vi "仪器电源管理.vi"() -> ()   [LabVIEW 2016, in "环境动力监测库.lvlib" / "G电源管理库.lvlib"]
uses:
  <vilib>/Utility/miscctls.llb/LVPointTypeDef.ctl
panel:
  in  "电源控制":T1
  in  "副屏看门狗启用":u16(ring) caption="副屏看门狗启用：" items=["关闭", "打开"]
  in  "副屏看门狗设置":u16 caption="副屏看门狗设置："
  out "副屏看门狗计时":u16 caption="副屏看门狗计时："
  in  "主屏看门狗启用":u16(ring) caption="主屏看门狗启用：" items=["关闭", "打开"]
  in  "主屏看门狗设置":u16 caption="主屏看门狗设置："
  out "主屏看门狗计时":u16 caption="主屏看门狗计时："
  # "仪器电源管理"
  # "s"
  # "s"
  # "s"
  # "s"
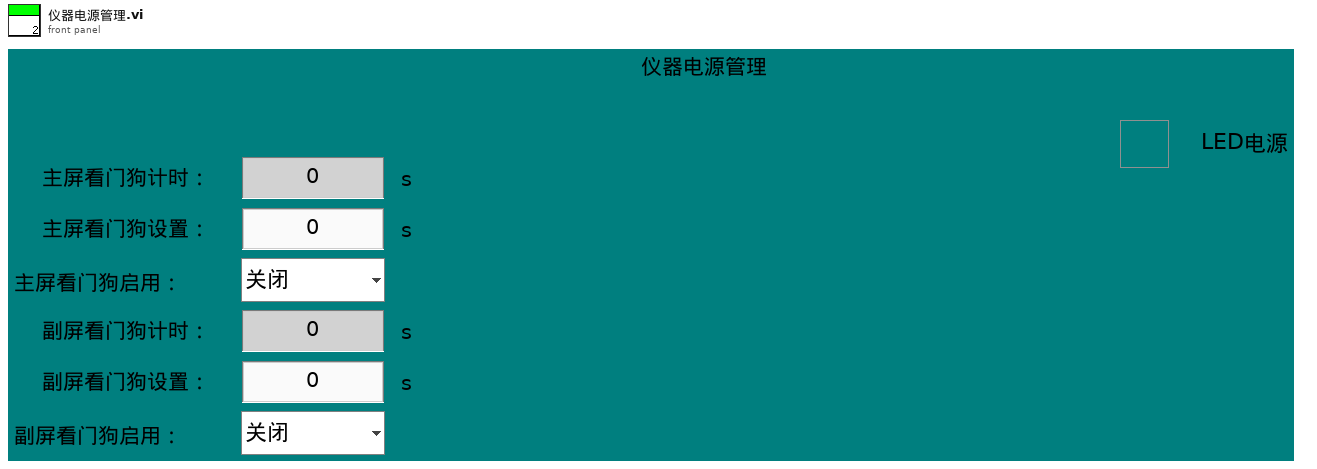
[diagram p1: front panel]
types:
  T1 = cluster{"氨氮电源":bool, "总磷电源":bool, "总氮电源":bool, "多参数电源":bool, "CODMn电源":bool, "CODCr电源":bool, "LED电源":bool}
  T2 = typedef "LVPointTypeDef.ctl" = cluster{"Horizontal":i16, "Vertical":i16}
  T3 = cluster{"采配水启用":bool, "CODMn启用":bool, "CODcr启用":bool, "氨氮启用":bool, "总磷启用":bool, "质控单元启用":bool, "流量计启用":bool, "电源管理启用":bool, "其他启用":bool, "多参数启用":bool, "超标留样启用":bool, "总氮启用":bool, "运行模式":enum16{"维护模式", "常规模式", "应急模式", "质控模式"}}
  T4 = cluster{"状态":cluster{"R0":i16, "R1":i16, "R2":i16, "R3":i16, "R4":i16, "R5":i16, "R6":i16, "R7":i16, "R8":i16, "R9":i16, "R10":i16, "R11":i16, "R12":i16, "R13":i16, "R14":i16, "R15":i16, "R16":i16, "R17":i16, "R18":i16, "R19":i16, "R20":i16, "R21":i16, "R22":i16, "R23":i16, "R24":i16, "R25":i16, "R26":i16, "R27":i16, "R28":i16, "R29":i16, "R30":i16, "R31":i16, "R32":i16, "R33":i16, "R34":i16, "R35":i16, "R36":i16, "R37":i16, "R38":i16, "R39":i16}, "输入状态":bool[], "输出状态":bool[], "参数设置":cluster{"R100":i16, "R101":i16, "R102":i16, "R103":i16, "R104":i16, "R105":i16, "R106":i16, "R107":i16, "R108":i16, "R109":i16, "R110":i16, "R111":i16, "R112":i16, "R113":i16, "R114":i16, "R115":i16, "R116":i16, "R117":i16, "R118":i16, "R119":i16, "R120":i16, "R121":i16, "R122":i16, "R123":i16}, "转换值":cluster{"AD0":sgl, "AD1":sgl, "AD2":sgl, "AD3":sgl, "AD4":sgl, "AD5":sgl}}
  T5 = cluster{"R100":i16, "R101":i16, "R102":i16, "R103":i16, "R104":i16, "R105":i16, "R106":i16, "R107":i16, "R108":i16, "R109":i16, "R110":i16, "R111":i16, "R112":i16, "R113":i16, "R114":i16, "R115":i16, "R116":i16, "R117":i16, "R118":i16, "R119":i16, "R120":i16, "R121":i16, "R122":i16, "R123":i16}
  T6 = cluster{"R0":i16, "R1":i16, "R2":i16, "R3":i16, "R4":i16, "R5":i16, "R6":i16, "R7":i16, "R8":i16, "R9":i16, "R10":i16, "R11":i16, "R12":i16, "R13":i16, "R14":i16, "R15":i16, "R16":i16, "R17":i16, "R18":i16, "R19":i16, "R20":i16, "R21":i16, "R22":i16, "R23":i16, "R24":i16, "R25":i16, "R26":i16, "R27":i16, "R28":i16, "R29":i16, "R30":i16, "R31":i16, "R32":i16, "R33":i16, "R34":i16, "R35":i16, "R36":i16, "R37":i16, "R38":i16, "R39":i16}
  T7 = cluster{"命令":string, "数据":cluster{"starting address":u16, "holding register values":u16[]}}
  T8 = cluster{"命令":string, "数据":cluster{"starting address":u16, "holding register value":u16}}
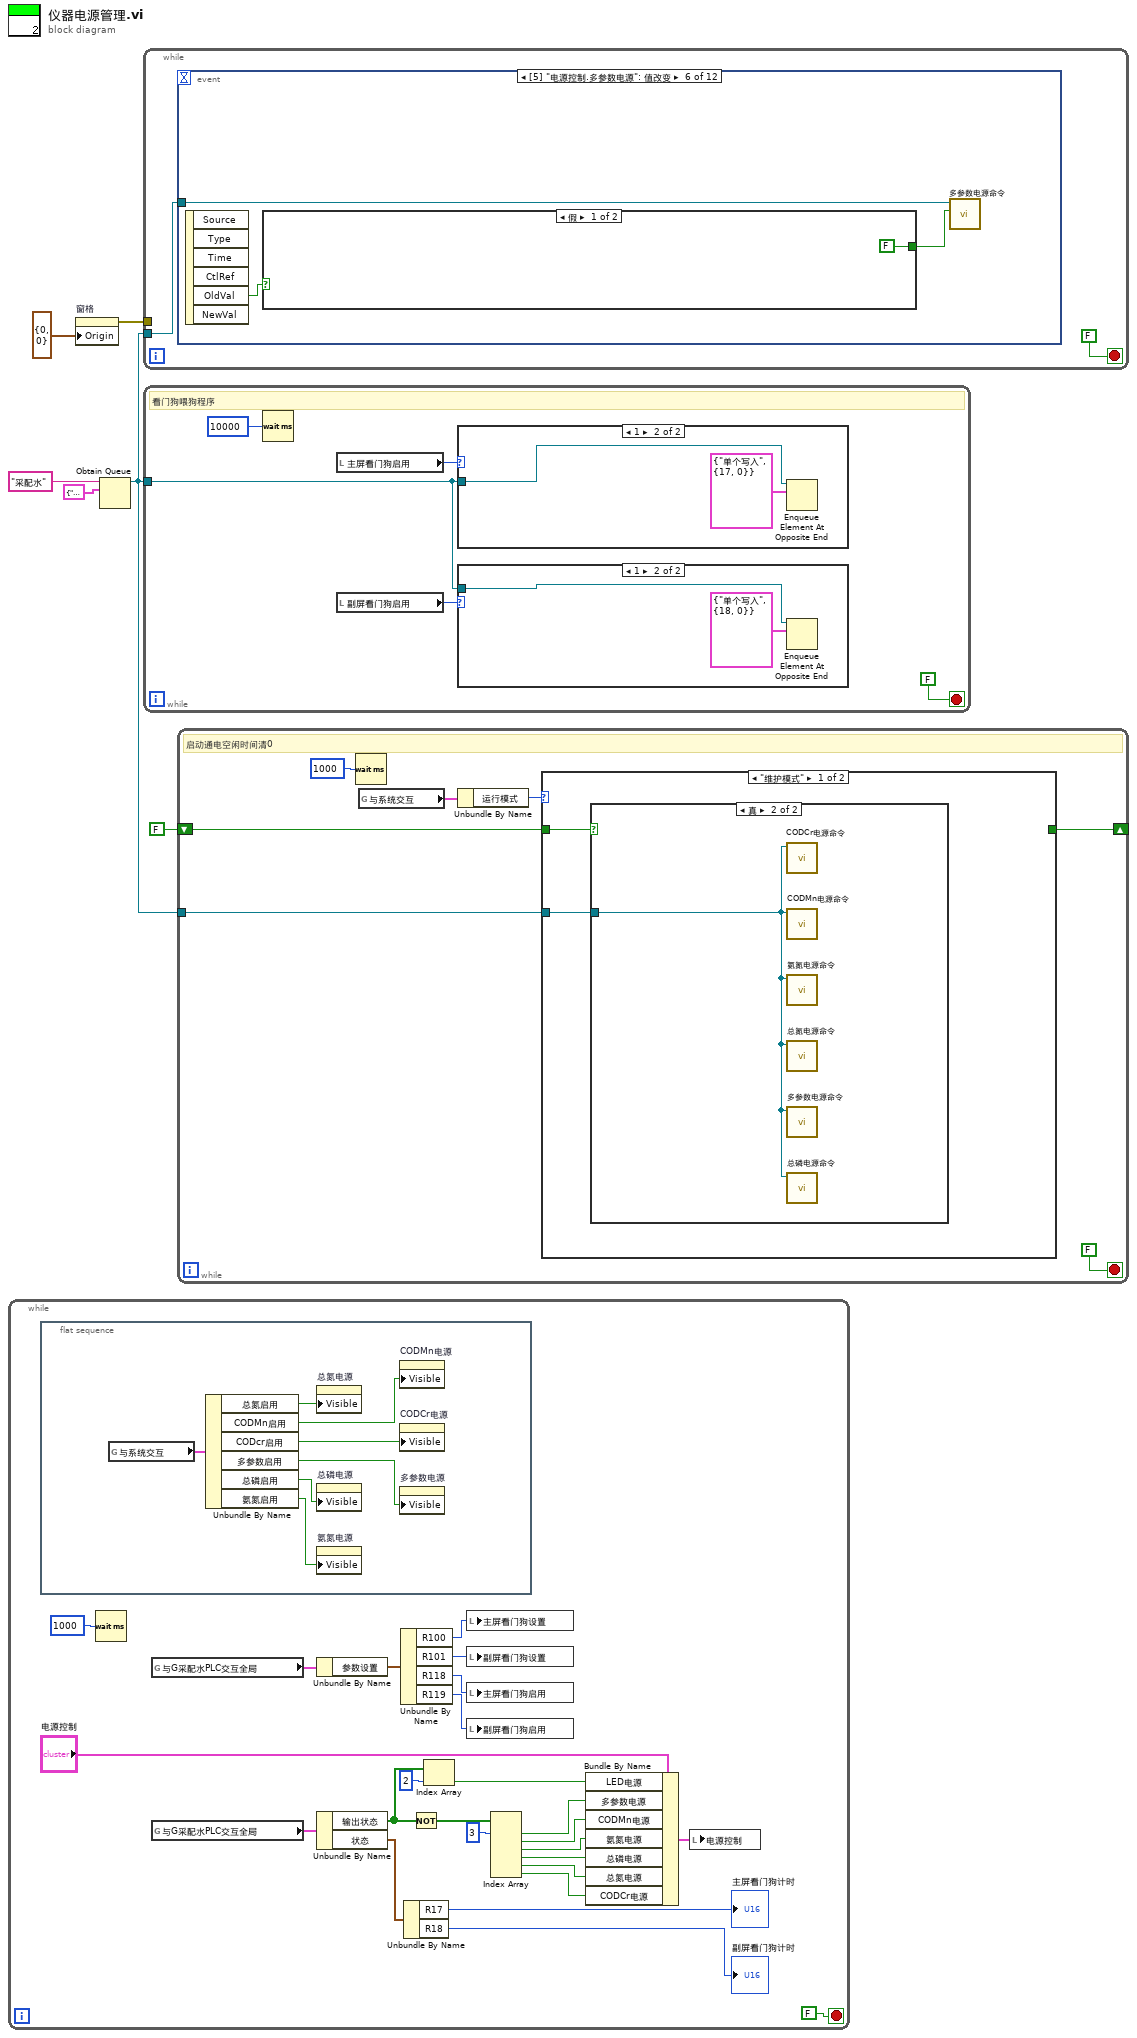
[diagram p0: block diagram]
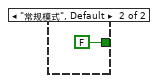
[diagram p5: hidden frame]
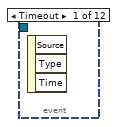
[diagram p6: hidden frame]
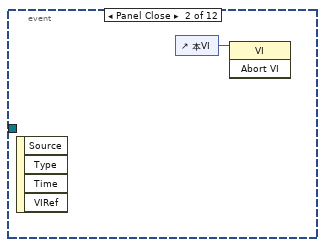
[diagram p7: hidden frame]
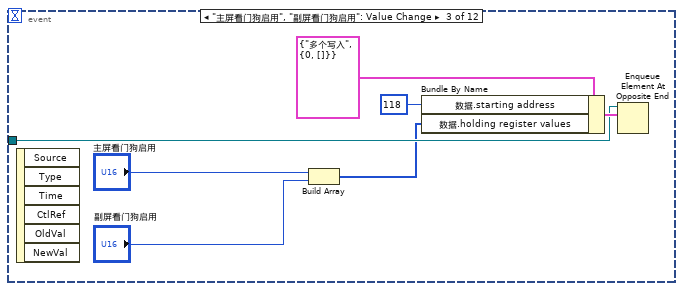
[diagram p8: hidden frame]
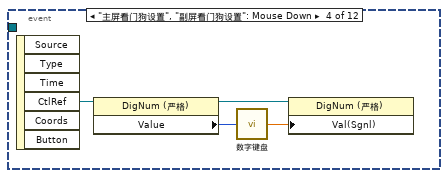
[diagram p9: hidden frame]
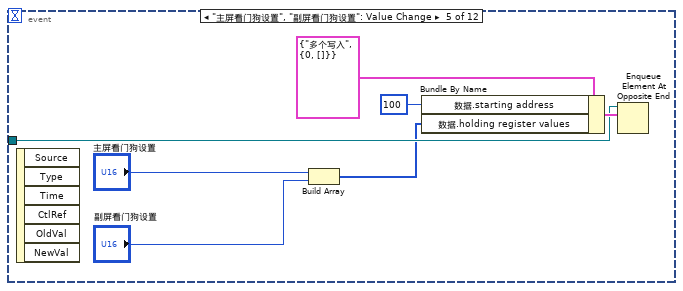
[diagram p10: hidden frame]
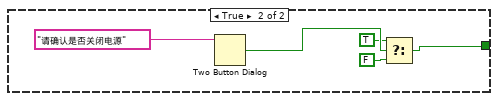
[diagram p11: hidden frame]
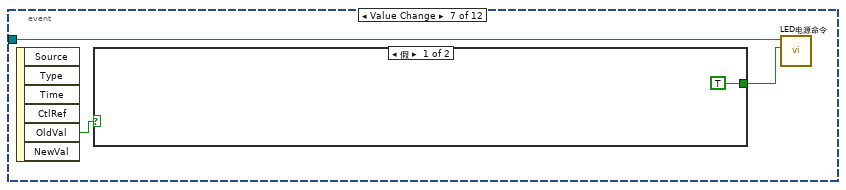
[diagram p12: hidden frame]
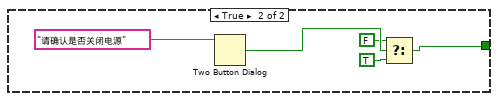
[diagram p13: hidden frame]
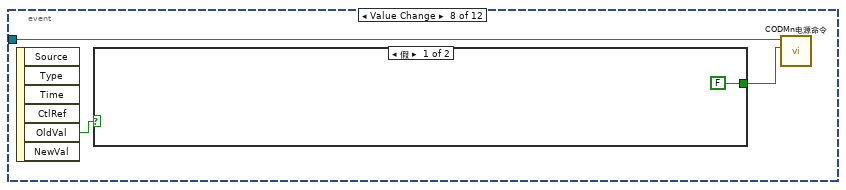
[diagram p14: hidden frame]
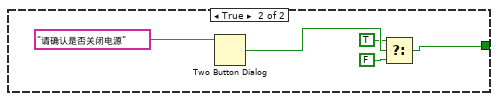
[diagram p15: hidden frame]
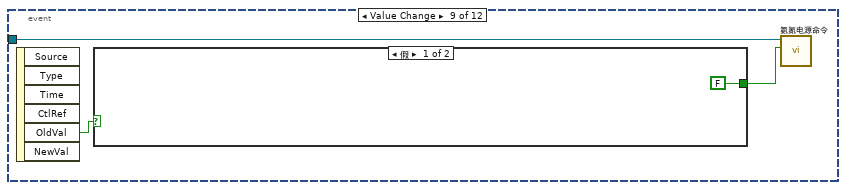
[diagram p16: hidden frame]
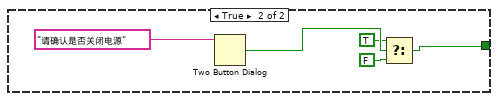
[diagram p17: hidden frame]
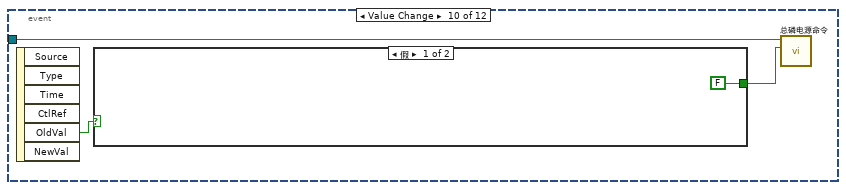
[diagram p18: hidden frame]
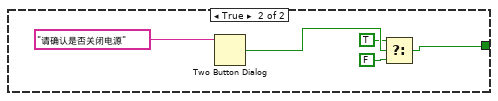
[diagram p19: hidden frame]
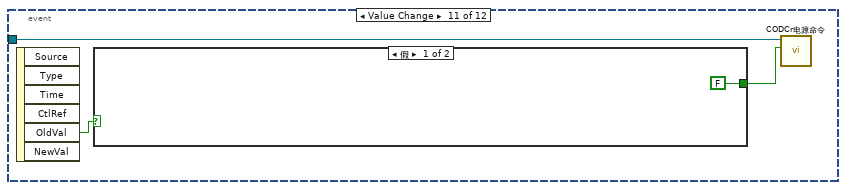
[diagram p20: hidden frame]
diagram:
  n1 = while {
    stop <- FALSE stop-if-true
    n2 = flat-sequence {
      frame #0 {
        n3 = global read "外部交互全局变量.vi" "与系统交互"() -> (w38:T3)
        n4 = Unbundle By Name(w38) -> ("总氮启用"=w37:bool, "CODMn启用"=w36:bool, "CODcr启用"=w32:bool, "多参数启用"=w33:bool, "总磷启用"=w34:bool, "氨氮启用"=w35:bool)
        n5 = property on="总氮电源" class="Bool (严格)"("Visible"=w37) -> ()  [unwired: 2 in, 2 out]
        n6 = property on="总磷电源" class="Bool (严格)"("Visible"=w34) -> ()  [unwired: 2 in, 2 out]
        n7 = property on="氨氮电源" class="Bool (严格)"("Visible"=w35) -> ()  [unwired: 2 in, 2 out]
        n8 = property on="CODMn电源" class="Bool (严格)"("Visible"=w36) -> ()  [unwired: 2 in, 2 out]
        n9 = property on="CODCr电源" class="Bool (严格)"("Visible"=w32) -> ()  [unwired: 2 in, 2 out]
        n10 = property on="多参数电源" class="Bool (严格)"("Visible"=w33) -> ()  [unwired: 2 in, 2 out]
      }
    }
    n11 = Wait (ms)(milliseconds to wait=u32 1000 ("等待时间（毫秒）")) -> ()  [unwired: 1 out]
    n12 = global read "外部交互全局变量.vi" "与G采配水PLC交互全局"() -> (w11:T4)
    n13 = global read "外部交互全局变量.vi" "与G采配水PLC交互全局"() -> (w9:T4)
    n14 = Unbundle By Name(w11) -> ("参数设置"=w10:T5)
    n15 = Unbundle By Name(w9) -> ("输出状态"=w8:bool[], "状态"=w7:T6)
    n16 = Unbundle By Name(w10) -> ("R100"=w26:i16, "R101"=w25:i16, "R118"=w24:i16, "R119"=w23:i16)
    n17 = Unbundle By Name(w7) -> ("R17"=→"主屏看门狗计时":i16, "R18"=→"副屏看门狗计时":i16)
    n18 = Not(x=w8) -> (.not. x?=w29:bool[])
    n19 = Index Array(array=w8, index=2 ("索引")) -> (element=w19:bool)
    n20 = local write "主屏看门狗设置"(w26) -> ()
    n21 = local write "副屏看门狗设置"(w25) -> ()
    n22 = local write "主屏看门狗启用"(w24) -> ()
    n23 = local write "副屏看门狗启用"(w23) -> ()
    n24 = Index Array(array=w29, index #1=3 ("索引")) -> (element #1=w18:bool, element #2=w17:bool, element #3=w16:bool, element #4=w15:bool, element #5=w14:bool, element #6=w13:bool)  [unwired: 5 in]
    n25 = Bundle By Name(cluster="电源控制", "LED电源"=w19, "多参数电源"=w18, "CODMn电源"=w17, "氨氮电源"=w16, "总磷电源"=w15, "总氮电源"=w14, "CODCr电源"=w13) -> (w12:T1)
    n26 = local write "电源控制"(w12) -> ()
  }
  n27 = property on="窗格" class="Pane"("Origin"=T2 {"Horizontal"=0, "Vertical"=0} ("原点")) -> (error out=w3:errorcluster)  [unwired: 2 in, 1 out]
  n28 = Obtain Queue(name (unnamed)="采配水" ("名称（未命名）"), element data type=cluster{"命令":string, "数据":variant} {"命令"="", "数据"=variant}) -> (queue out=w1:refnum<queue>)  [unwired: 3 in, 2 out]
  n29 = while {
    tunnel: w1 -> [w40]
    tunnel: w3 -> [_]
    stop <- FALSE stop-if-true
    n30 = event shown="[5] \"电源控制.多参数电源\": 值改变" {
      selector: _ -> [_ _ _ _ _ _ _ _ _ _ _ _]
      dyn-events: _ -> [_ _ _ _ _ _ _ _ _ _ _ _]
      timeout: _ -> [_ _ _ _ _ _ _ _ _ _ _ _]
      tunnel: w40 -> [_ _ w45 _ w56 w62 w70 w80 w89 w98 w107 w116]
      event Timeout {
        n31 = event-data() -> ()  [unwired: 1 in, 3 out]
      }
      event Panel Close {
        n32 = event-data() -> ()  [unwired: 1 in, 4 out]
        n33 = control-ref of="本VI"() -> (w41:refnum<vi>)
        n34 = invoke class="VI" method="Abort VI"(reference=w41) -> ()  [unwired: 2 in, 3 out]
      }
      event "主屏看门狗启用", "副屏看门狗启用": Value Change {
        n35 = event-data() -> ()  [unwired: 1 in, 6 out]
        n36 = Build Array("主屏看门狗启用", "副屏看门狗启用") -> (w42:u16[])
        n37 = Bundle By Name(cluster=T7 {"命令"="多个写入", "数据"={"starting address"=0, "holding register values"=[]}} ("元素"), "数据.starting address"=u16 118, "数据.holding register values"=w42) -> (w46:T7)
        n38 = Enqueue Element At Opposite End(queue=w45, element=w46) -> ()  [unwired: 2 in, 3 out]
      }
      event "主屏看门狗设置", "副屏看门狗设置": Mouse Down {
        n39 = event-data() -> ("CtlRef"=w49:refnum<vi>)  [unwired: 1 in, 5 out]
        n40 = property class="DigNum (严格)"(reference=w49) -> (reference out=w51:refnum<vi>, "Value"=w52:u16)  [unwired: 1 in, 1 out]
        n41 = call "数字键盘.vi"("OldNumber"=w52) -> ("NewNumber"=w50:sgl)
        n42 = property class="DigNum (严格)"(reference=w51, "Val(Sgnl)"=w50) -> ()  [unwired: 1 in, 2 out]
      }
      event "主屏看门狗设置", "副屏看门狗设置": Value Change {
        n43 = event-data() -> ()  [unwired: 1 in, 6 out]
        n44 = Build Array("主屏看门狗设置", "副屏看门狗设置") -> (w53:u16[])
        n45 = Bundle By Name(cluster=T7 {"命令"="多个写入", "数据"={"starting address"=0, "holding register values"=[]}} ("元素"), "数据.starting address"=u16 100, "数据.holding register values"=w53) -> (w57:T7)
        n46 = Enqueue Element At Opposite End(queue=w56, element=w57) -> ()  [unwired: 2 in, 3 out]
      }
      event "电源控制.多参数电源": Value Change {
        n47 = event-data() -> ("OldVal"=w61:bool)  [unwired: 1 in, 5 out]
        n48 = case shown="假" w61 {
          tunnel: [FALSE ("T button?") w64] -> w60
          frame False {
          }
          frame True {
            n49 = Two Button Dialog(message="请确认是否关闭电源" ("消息")) -> (T button?=w67:bool)  [unwired: 2 in]
            n50 = Select(t=TRUE, s=w67, f=FALSE ("T button?")) -> (s? t:f=w64:bool)
          }
        }
        n51 = call "多参数电源命令.vi"("通电/断电"=w60, "队列"=w62) -> ()  [unwired: 9 in, 1 out]
      }
      event "电源控制.LED电源": Value Change {
        n52 = event-data() -> ("OldVal"=w71:bool)  [unwired: 1 in, 5 out]
        n53 = case shown="假" w71 {
          tunnel: [TRUE ("T button?") w73] -> w69
          frame False {
          }
          frame True {
            n54 = Two Button Dialog(message="请确认是否关闭电源" ("消息")) -> (T button?=w76:bool)  [unwired: 2 in]
            n55 = Select(t=FALSE, s=w76, f=TRUE ("T button?")) -> (s? t:f=w73:bool)
          }
        }
        n56 = call "LED电源命令.vi"("通电/断电"=w69, "队列"=w70) -> ()  [unwired: 9 in, 1 out]
      }
      event "电源控制.CODMn电源": Value Change {
        n57 = event-data() -> ("OldVal"=w79:bool)  [unwired: 1 in, 5 out]
        n58 = case shown="假" w79 {
          tunnel: [FALSE ("T button?") w82] -> w78
          frame False {
          }
          frame True {
            n59 = Two Button Dialog(message="请确认是否关闭电源" ("消息")) -> (T button?=w85:bool)  [unwired: 2 in]
            n60 = Select(t=TRUE, s=w85, f=FALSE ("T button?")) -> (s? t:f=w82:bool)
          }
        }
        n61 = call "CODMn电源命令.vi"("通电/断电"=w78, "队列"=w80) -> ()  [unwired: 9 in, 1 out]
      }
      event "电源控制.氨氮电源": Value Change {
        n62 = event-data() -> ("OldVal"=w88:bool)  [unwired: 1 in, 5 out]
        n63 = case shown="假" w88 {
          tunnel: [FALSE ("T button?") w91] -> w87
          frame False {
          }
          frame True {
            n64 = Two Button Dialog(message="请确认是否关闭电源" ("消息")) -> (T button?=w94:bool)  [unwired: 2 in]
            n65 = Select(t=TRUE, s=w94, f=FALSE ("T button?")) -> (s? t:f=w91:bool)
          }
        }
        n66 = call "氨氮电源命令.vi"("通电/断电"=w87, "队列"=w89) -> ()  [unwired: 9 in, 1 out]
      }
      event "电源控制.总磷电源": Value Change {
        n67 = event-data() -> ("OldVal"=w97:bool)  [unwired: 1 in, 5 out]
        n68 = case shown="假" w97 {
          tunnel: [FALSE ("T button?") w100] -> w96
          frame False {
          }
          frame True {
            n69 = Two Button Dialog(message="请确认是否关闭电源" ("消息")) -> (T button?=w103:bool)  [unwired: 2 in]
            n70 = Select(t=TRUE, s=w103, f=FALSE ("T button?")) -> (s? t:f=w100:bool)
          }
        }
        n71 = call "总磷电源命令.vi"("通电/断电"=w96, "队列"=w98) -> ()  [unwired: 9 in, 1 out]
      }
      event "电源控制.CODCr电源": Value Change {
        n72 = event-data() -> ("OldVal"=w106:bool)  [unwired: 1 in, 5 out]
        n73 = case shown="假" w106 {
          tunnel: [FALSE ("T button?") w109] -> w105
          frame False {
          }
          frame True {
            n74 = Two Button Dialog(message="请确认是否关闭电源" ("消息")) -> (T button?=w112:bool)  [unwired: 2 in]
            n75 = Select(t=TRUE, s=w112, f=FALSE ("T button?")) -> (s? t:f=w109:bool)
          }
        }
        n76 = call "CODCr电源命令.vi"("通电/断电"=w105, "队列"=w107) -> ()  [unwired: 9 in, 1 out]
      }
      event "电源控制.总氮电源": Value Change {
        n77 = event-data() -> ("OldVal"=w114:bool)  [unwired: 1 in, 5 out]
        n78 = case shown="假" w114 {
          tunnel: [FALSE ("T button?") w118] -> w115
          frame False {
          }
          frame True {
            n79 = Two Button Dialog(message="请确认是否关闭电源" ("消息")) -> (T button?=w121:bool)  [unwired: 2 in]
            n80 = Select(t=TRUE, s=w121, f=FALSE ("T button?")) -> (s? t:f=w118:bool)
          }
        }
        n81 = call "总氮电源命令.vi"("通电/断电"=w115, "队列"=w116) -> ()  [unwired: 9 in, 1 out]
      }
    }
  }
  n82 = while {
    tunnel: w1 -> [w127]
    stop <- FALSE stop-if-true
    # "看门狗喂狗程序"
    n83 = Wait (ms)(milliseconds to wait=u32 10000 ("等待时间（毫秒）")) -> ()  [unwired: 1 out]
    n84 = local read "主屏看门狗启用"() -> (w126:u16)
    n85 = local read "副屏看门狗启用"() -> (w125:u16)
    n86 = case shown="1" w126 {
      tunnel: w127 -> [_ w130]
      frame 0, Default {
      }
      frame 1 {
        n87 = Enqueue Element At Opposite End(queue=w130, element=T8 {"命令"="单个写入", "数据"={"starting address"=17, "holding register value"=0}} ("元素")) -> ()  [unwired: 2 in, 3 out]
      }
    }
    n88 = case shown="1" w125 {
      tunnel: w127 -> [_ w128]
      frame 0, Default {
      }
      frame 1 {
        n89 = Enqueue Element At Opposite End(queue=w128, element=T8 {"命令"="单个写入", "数据"={"starting address"=18, "holding register value"=0}} ("元素")) -> ()  [unwired: 2 in, 3 out]
      }
    }
  }
  n90 = while {
    tunnel: w1 -> [w136]
    shift-right: [w134] -> _
    shift-left: FALSE -> [w135]
    stop <- FALSE stop-if-true
    # "启动通电空闲时间清0"
    n91 = Wait (ms)(milliseconds to wait=u32 1000 ("等待时间（毫秒）")) -> ()  [unwired: 1 out]
    n92 = global read "外部交互全局变量.vi" "与系统交互"() -> (w133:T3)
    n93 = Unbundle By Name(w133) -> ("运行模式"=w132:enum16{"维护模式", "常规模式", "应急模式", "质控模式"})
    n94 = case shown="\"维护模式\"" w132 {
      tunnel: w136 -> [w140 _]
      tunnel: w135 -> [w139 _]
      tunnel: [_ FALSE] -> w134
      frame "维护模式" {
        n95 = case shown="真" w139 {
          tunnel: w140 -> [_ w141]
          frame False {
          }
          frame True {
            n96 = call "CODCr电源命令.vi"("队列"=w141) -> ()  [unwired: 10 in, 1 out]
            n97 = call "CODMn电源命令.vi"("队列"=w141) -> ()  [unwired: 10 in, 1 out]
            n98 = call "氨氮电源命令.vi"("队列"=w141) -> ()  [unwired: 10 in, 1 out]
            n99 = call "总氮电源命令.vi"("队列"=w141) -> ()  [unwired: 10 in, 1 out]
            n100 = call "多参数电源命令.vi"("队列"=w141) -> ()  [unwired: 10 in, 1 out]
            n101 = call "总磷电源命令.vi"("队列"=w141) -> ()  [unwired: 10 in, 1 out]
          }
        }
      }
      frame "常规模式", Default {
      }
    }
  }
